vi "Test Debug Corner Case.vi"(11 "Test Case In":refnum<class "Added Section Finder Test.lvclass">) -> (0 "error out":errorcluster, 3 "Test Case Out":refnum<class "Added Section Finder Test.lvclass">)   [LabVIEW 2020, in "Added Section Finder Test.lvclass"]
uses:
  Added Section Finder Test.lvclass
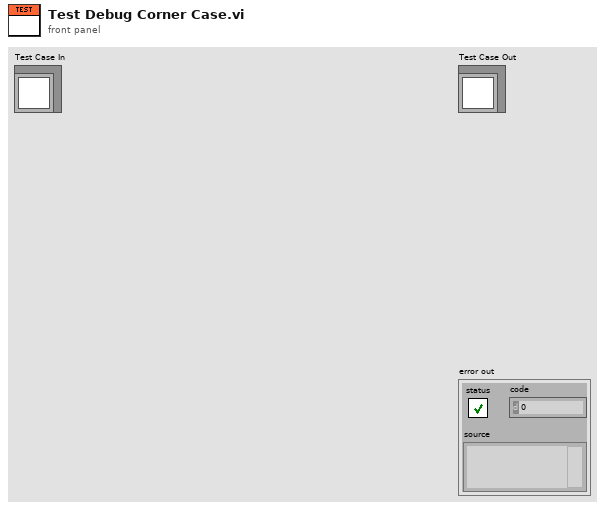
[diagram p1: front panel]
types:
  T1 = cluster{"Selection Start":u32, "Selection End":u32}
  T2 = cluster{"Selection Start":u32, "Selection End":u32}[]
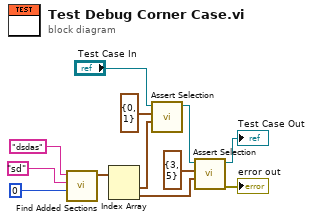
[diagram p0: block diagram]
diagram:
  n1 = call "Find Added Sections.vi"("Offset"=u32 0 ("Index"), "Reference"="sd", "Target"="dsdas") -> ("Sections in Target"=w8:T2)  [unwired: 8 in]
  n2 = Index Array(array=w8) -> (element #1=w4:T1, element #2=w5:T1)  [unwired: 2 in]
  n3 = call "Assert Selection.vi"("Actual"=w4, "Expected"=T1 {"Selection Start"=0, "Selection End"=1} ("Text.Selection"), "Added Section Finder Test In"="Test Case In") -> ("Added Section Finder Test Out"=w7:refnum<class "Added Section Finder Test.lvclass">)  [unwired: 7 in, 1 out]
  n4 = call "Assert Selection.vi"("Actual"=w5, "Expected"=T1 {"Selection Start"=3, "Selection End"=5} ("Text.Selection"), "Added Section Finder Test In"=w7) -> ("error out"=→"error out":errorcluster, "Added Section Finder Test Out"=→"Test Case Out":refnum<class "Added Section Finder Test.lvclass">)  [unwired: 7 in]
